vi "PXI-2512.Async.vi"(10 "Parameters":variant, 11 "Process":refnum<class "Process.lvclass">) -> ()   [LabVIEW 2020, in "PXI-2512 Engine.lvlib"]
uses:
  PXI-2512 Engine.lvlib
  <vilib>/NI/NIVS Inline Async API/_VS Inline Async API/Process/Process.lvclass
  <vilib>/NI/NIVS Inline Async API/_Data Access Engine/Data Access Engine/Data Access Engine.lvclass
  Shared/Compiled.Settings.ctl
  Shared/PXI-2512 Shared.lvlib
  <instrlib>/niSwitch/niSwitch.llb/niSwitch Topologies.ctl
  <vilib>/NI/NIVS Inline Async API/_Data Access Engine/Data Access Engine/Methods/Read.Data.vi
  <vilib>/NI/NIVS Inline Async API/_Data Access Engine/Data Access Engine/Methods/Write.Data.vi
  <vilib>/NI/NIVS Inline Async API/_Data Access Engine/Data Access Engine/Methods/Read.Lookup.vi
  <vilib>/NI/NIVS Inline Async API/_Data Access Engine/Data Access Engine/Methods/Write.Lookup.vi
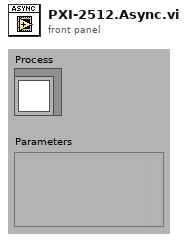
[diagram p1: front panel]
types:
  T1 = typedef "niSwitch Topologies.ctl" = string
  T2 = typedef "PXI-2512 Shared.lvlib/Compiled.Settings.ctl" = cluster{"Name":string, "Async Init Timeout":u16, "Hardware Device Name":string}
  T3 = typedef "Data Access Engine.lvlib/Data Access Engine.lvclass/Write.DVR.ctl" = refnum<data-value>
  T4 = typedef "Data Access Engine.lvlib/Data Access Engine.lvclass/Read.DVR.ctl" = refnum<data-value>
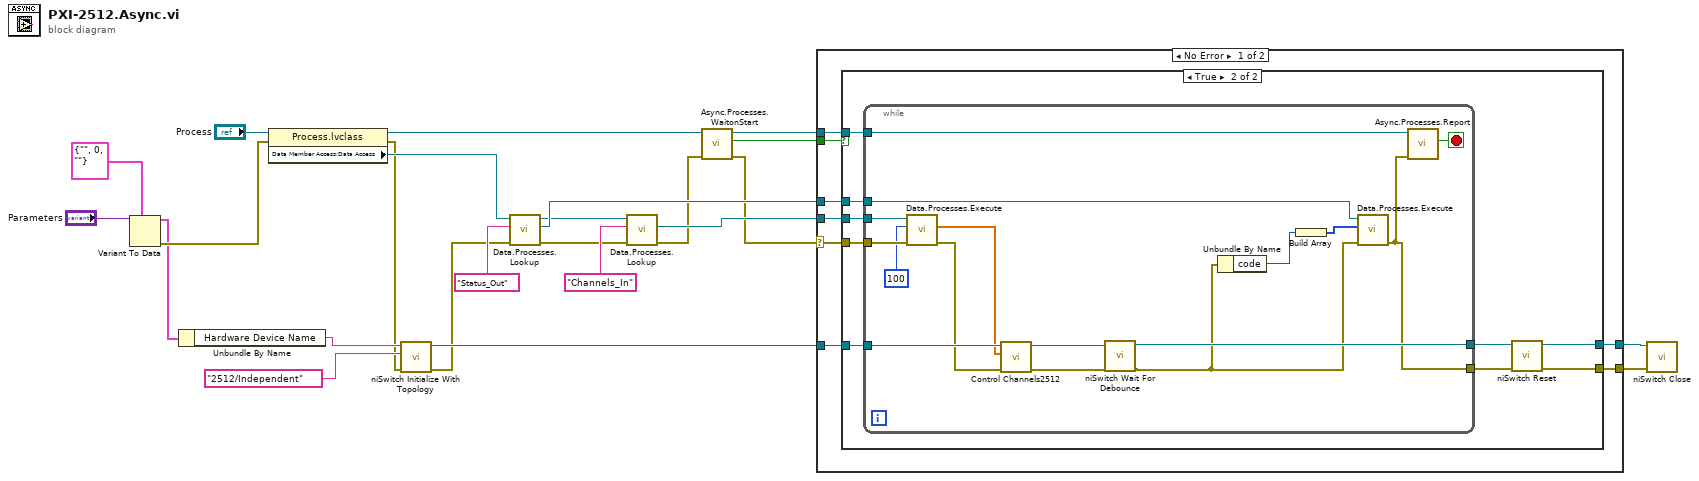
[diagram p0: block diagram]
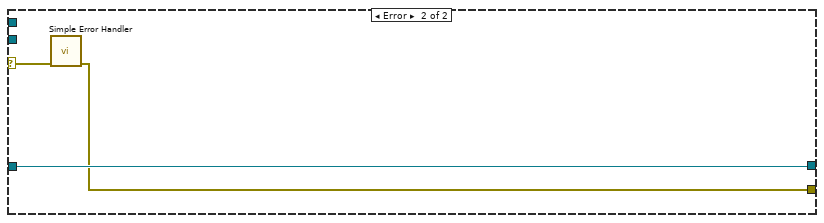
[diagram p3: hidden frame]
diagram:
  n1 = Variant To Data(type=T2 {"Name"="", "Async Init Timeout"=0, "Hardware Device Name"=""} ("Compiled.Settings"), Variant="Parameters") -> (data=w9:T2, error out=w10:errorcluster)  [unwired: 1 in]
  n2 = Unbundle By Name(w9) -> ("Hardware Device Name"=w8:string)
  n3 = property class="Process.lvclass"(reference="Process", error in=w10) -> (reference out=w14:refnum<class "Process.lvclass">, error out=w6:errorcluster, "Data Member Access:Data Access"=w13:refnum<class "Data Access Engine.lvclass">)
  n4 = call <instrlib>:"niSwitch Initialize With Topology.vi"("error in (no error)"=w6, "topology name"=T1 "2512/Independent", "resource name"=w8) -> ("error out"=w2:errorcluster, "instrument handle out"=w5:refnum<k15>)  [unwired: 7 in]
  n5 = call-poly <vilib>:"Data.Processes.Lookup.vi"("error in (no error)"=w2, "Name"="Status_Out", "Data Access API in"=w13) -> ("error out"=w19:errorcluster, "Ref"=w18:T3, "Data Access API out"=w17:refnum<class "Data Access Engine.lvclass">)  [unwired: 5 in, 1 out]
  n6 = call-poly <vilib>:"Data.Processes.Lookup.vi"("error in (no error)"=w19, "Name"="Channels_In", "Data Access API in"=w17) -> ("error out"=w16:errorcluster, "Ref"=w21:T4)  [unwired: 5 in, 2 out]
  n7 = call <vilib>:"Async.Processes.WaitonStart.vi"("error in (no error)"=w16, "Process"=w14) -> ("error out"=w1:errorcluster, "Execute"=w24:bool, "Process out"=w23:refnum<class "Process.lvclass">)  [unwired: 7 in]
  n8 = case shown="No Error" w1 {
    selector: w1 -> [w28 w62]
    tunnel: w24 -> [w32 _]
    tunnel: w23 -> [w31 _]
    tunnel: w18 -> [w30 _]
    tunnel: w21 -> [w29 _]
    tunnel: w5 -> [w27 w61]
    tunnel: [w26 w61] -> w4
    tunnel: [w25 w60] -> w3
    frame No Error {
      n9 = case shown="True" w32 {
        tunnel: w28 -> [w33 w40]
        tunnel: w31 -> [_ w41]
        tunnel: w29 -> [_ w43]
        tunnel: w30 -> [_ w42]
        tunnel: w27 -> [w34 w39]
        tunnel: [w34 w36] -> w26
        tunnel: [w33 w35] -> w25
        frame False {
        }
        frame True {
          n10 = while {
            tunnel: w40 -> [w55]
            tunnel: w41 -> [w59]
            tunnel: w43 -> [w57]
            tunnel: w42 -> [w56]
            tunnel: w39 -> [w53]
            tunnel: [w46] -> w38
            tunnel: [w44] -> w37
            stop <- w58 stop-if-true
            n11 = call-poly <vilib>:"Data.Processes.Execute.vi"("error in (no error)"=w55, "timeout ms"=100, "Ref"=w57) -> ("error out"=w52:errorcluster, "Values"=w51:dbl[])  [unwired: 6 in, 1 out]
            n12 = call "Control Channels2512.vi"("error in (no error)"=w52, "Values"=w51, "IVI Refnum in"=w53) -> ("error Out"=w47:errorcluster, "IVI Refnum out"=w48:refnum<k15>)  [unwired: 7 in]
            n13 = call <instrlib>:"niSwitch Wait For Debounce.vi"("error in (no error)"=w47, "instrument handle"=w48) -> ("error out"=w45:errorcluster, "instrument handle out"=w46:refnum<k15>)  [unwired: 8 in]
            n14 = Unbundle By Name(w45) -> ("code"=w50:i32)
            n15 = Build Array(w50) -> (w49:i32[])
            n16 = call-poly <vilib>:"Data.Processes.Execute.vi"("error in (no error)"=w45, "Values"=w49, "Ref"=w56) -> ("error out"=w44:errorcluster)  [unwired: 8 in]
            n17 = call <vilib>:"Async.Processes.Report.vi"("Error"=w44, "Process in"=w59) -> ("Stop"=w58:bool)  [unwired: 8 in, 1 out]
          }
          n18 = call <instrlib>:"niSwitch Reset.vi"("error in (no error)"=w37, "instrument handle"=w38) -> ("error out"=w35:errorcluster, "instrument handle out"=w36:refnum<k15>)  [unwired: 8 in]
        }
      }
    }
    frame Error {
      n19 = call <vilib>:"Simple Error Handler.vi"("error in (no error)"=w62) -> ("error out"=w60:errorcluster)  [unwired: 4 in, 4 out]
    }
  }
  n20 = call <instrlib>:"niSwitch Close.vi"("error in (no error)"=w3, "instrument handle"=w4) -> ()  [unwired: 9 in, 1 out]
